vi "1kclass_10dt.vi"() -> (0 "max jitter (uS)":dbl format="%.2f", 1 "mean time (uS)":dbl format="%.2f", 2 "standard deviation (uS)":dbl format="%.2f", 3 "execution histogram":T1(graph), 4 "Error":errorcluster, 5 "execution times (uS)":dbl[](graph))   [LabVIEW 2013]
uses:
  <vilib>/platform/TimedLoop/XDataNode/XDataNode.xnode
  <vilib>/Platform/TimedLoop/XDataNode/nitl_modes.ctl
  <vilib>/Platform/TimedLoop/XDataNode/XDNodeRunTimeDep.lvlib
  <vilib>/Platform/TimedLoop/XDataNode/wakeup.ctl
  <vilib>/Platform/TimedLoop/XDataNode/timing_clust.ctl
  standard timing source/ms timing source.lvclass
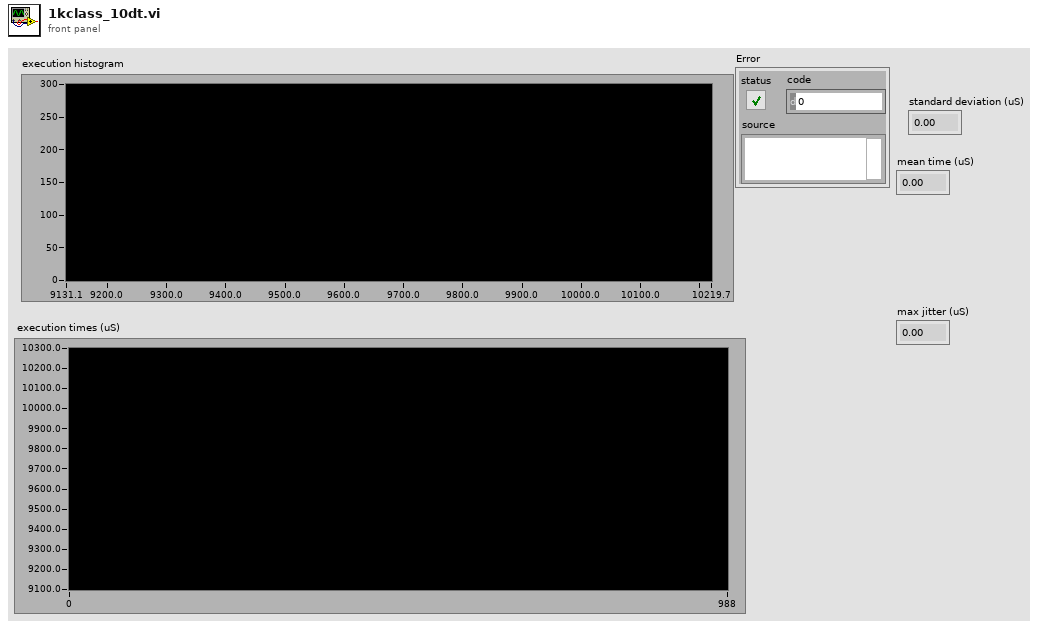
[diagram p1: front panel]
types:
  T1 = cluster{"X Values":dbl[], "Histogram: h(x)":i32[]}
  T2 = typedef "XDNodeRunTimeDep.lvlib/timing_clust.ctl" = cluster{"Expected End [f-1]":u64, "Actual End [f-1]":u64, "Finished Late? [f-1]":bool, "Expected End [i-1]":u64, "Actual End [i-1]":u64, "Finished Late? [i-1]":bool, "Expected Start [i]":u64, "Actual Start [i]":u64, "Expected Start [f]":u64, "Actual Start [f]":u64, "Source Name":string, "Structure Name":string, "Period":i64, "Deadline":i64, "Offset":i64, "Start":i64, "Priority":i32, "Timeout":i32, "Mode":T3, "Wakeup Reason":T4, "Error":errorcluster, "Source Type":string, "Secondary Source Type":string, "Global End Time":u64, "Global Start Time":u64, "Frame Duration":u64, "Iteration Duration":u64, "Assigned CPU":i32, "I/O Scan Engine Mode":u32}
  T3 = typedef "XDNodeRunTimeDep.lvlib/nitl_modes.ctl" = enum32{"No Change", "Process missed periods, maintain original phase", "Discard missed periods, maintain original phase", "Process missed periods, ignore original phase", "Discard missed periods, ignore original phase"}
  T4 = typedef "XDNodeRunTimeDep.lvlib/wakeup.ctl" = enum32{"Normal", "Aborted", "Asynchronous wakeup", "Timing source error", "Timed loop error", "Timeout"}
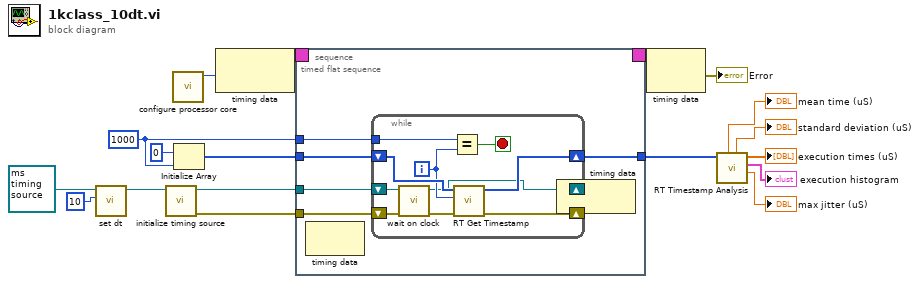
[diagram p0: block diagram]
diagram:
  w16 = 1000 ("x")
  n1 = call "set dt.vi"("dt"=u32 10, "timing source in"=refnum<class "ms timing source.lvclass"> refnum ("ms timing source.lvclass")) -> ("timing source out"=w4:refnum<class "ms timing source.lvclass">)  [unwired: 9 in]
  n2 = call-dynamic "initialize timing source.vi"("timing source in"=w4) -> ("error out"=w2:errorcluster, "timing source out"=w3:refnum<class "ms timing source.lvclass">)  [unwired: 9 in]
  n3 = call "configure processor core.vi"() -> ("Processor"=w6:i32)  [unwired: 11 in]
  n4 = Initialize Array(u64 0, w16) -> (w17:u64[])
  n5 = node-c288(w6) -> (w9:T2)
  n6 = timed-sequence {
    timing: w9 -> [_]
    timing-out: [_] -> w8
    tunnel: w16 -> [w23]
    tunnel: w17 -> [w22]
    tunnel: [w21] -> w15
    tunnel: w3 -> [w20]
    tunnel: w2 -> [w19]
    n7 = timed-flat-sequence {
      tunnel: w23 -> [w28]
      tunnel: w22 -> [w27]
      tunnel: [w26] -> w21
      tunnel: w20 -> [w25]
      tunnel: w19 -> [w24]
      n8 = node-c288() -> ()  [unwired: 1 in, 1 out]
      n9 = while {
        tunnel: w28 -> [w38]
        shift-right: [w36] -> w26
        shift-left: w27 -> [w37]
        shift-right: [w31] -> _
        shift-left: w25 -> [w32]
        shift-right: [w30] -> _
        shift-left: w24 -> [w29]
        i -> [w34]
        stop <- w35 stop-if-true
        n10 = call-dynamic "wait on clock.vi"("error in"=w29, "timing source in"=w32) -> ("error out"=w33:errorcluster, "timing source out"=w31:refnum<class "ms timing source.lvclass">)  [unwired: 7 in, 1 out]
        n11 = Equal?(x=w38, y=w34) -> (x = y?=w35:bool)
        n12 = call <vilib>:"RT Get Timestamp.vi"("error in (no error)"=w33, "iteration"=w34, "timestamp array in"=w37) -> ("error out"=w30:errorcluster, "timestamp array out"=w36:u64[])  [unwired: 7 in]
      }
      n13 = node-c288() -> ()  [unwired: 1 in, 1 out]
    }
  }
  n14 = node-c288(w8) -> (→"Error":errorcluster)
  n15 = call <vilib>:"RT Timestamp Analysis.vi"("timestamp array"=w15) -> ("max jitter (uS)"=→"max jitter (uS)":dbl, "execution histogram"=→"execution histogram":T1, "execution times (uS)"=→"execution times (uS)":dbl[], "standard deviation (uS)"=→"standard deviation (uS)":dbl, "mean time (uS)"=→"mean time (uS)":dbl)  [unwired: 5 in, 1 out]
